vi "optagefrekvenssignal0.8.vi"() -> ()   [LabVIEW 2014]
uses:
  <vilib>/measure/maspectr.llb/FFT Power Spectrum and PSD for 1 Chan.vi
  <vilib>/Utility/file.llb/Write To Spreadsheet File (DBL).vi
  <vilib>/measure/NI_MAPro.lvlib
panel:
  out "Resonansfrekvens, første 10 målinger":dbl[](array[numeric])
  in  "Tid(sek)":dbl
  out "Resonansfrekvens af kammer med objekt":dbl
  out "FFT af lydsignal":dbl[](graph)
  out "Lydsignal":waveform(dbl)(graph)
  # "Gennemsnit"
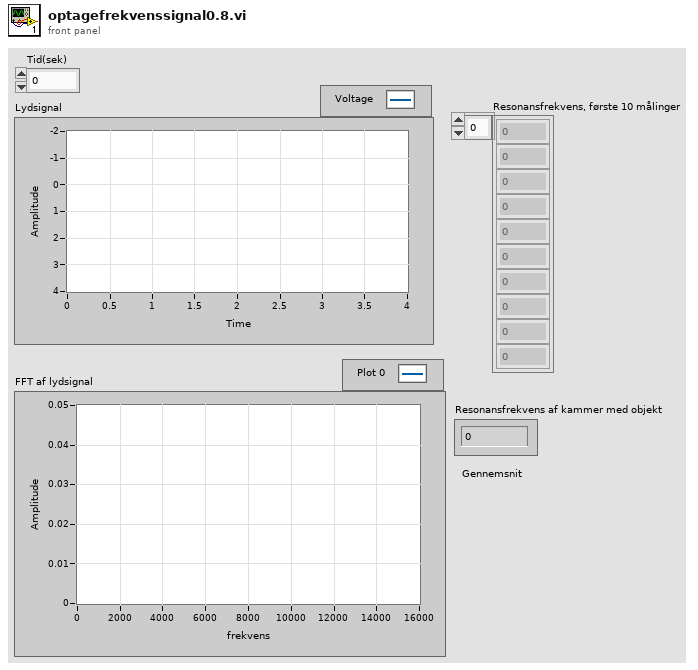
[diagram p1: front panel]
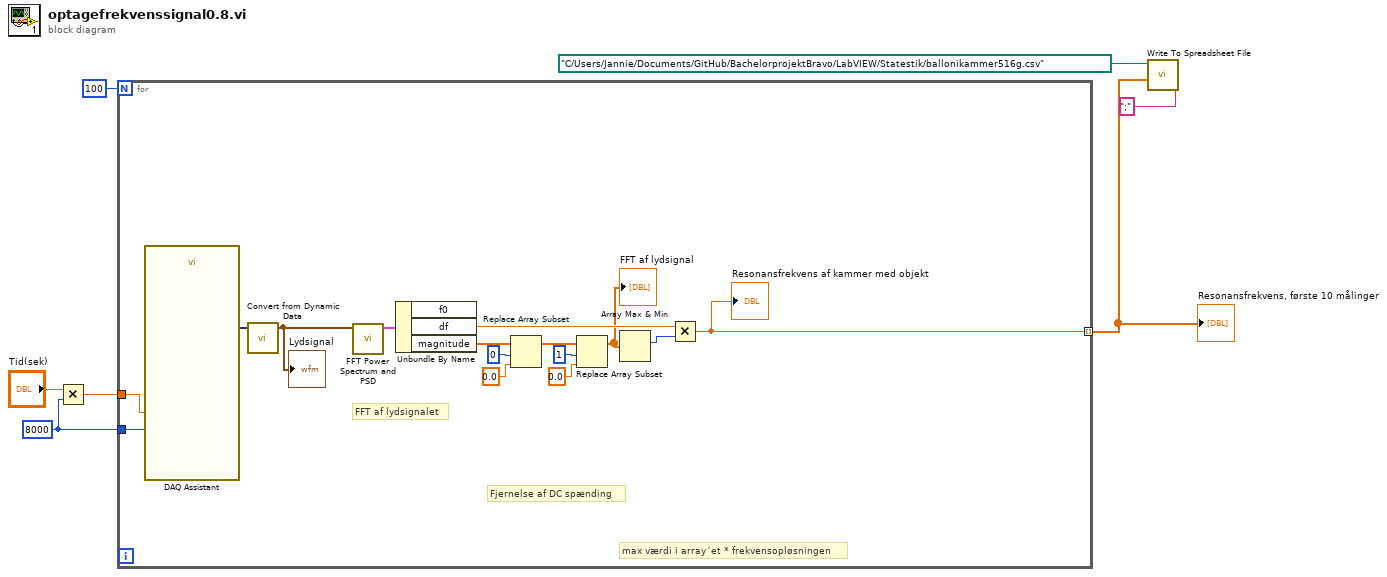
[diagram p0: block diagram]
diagram:
  w3 = 8000
  n1 = Multiply(x="Tid(sek)", y=w3) -> (x*y=w2:dbl)
  n2 = for {
    N: 100 -> [_]
    tunnel: [w12] -> w1 mode=indexing
    tunnel: w3 -> [w10]
    tunnel: w2 -> [w9]
    # "max værdi i array´et * frekvensopløsningen"
    # "Fjernelse af DC spænding"
    # "FFT af lydsignalet"
    n3 = call "DAQ Assistant"("rate"=w10, "number of samples"=w9) -> ("data"=w8:dynamicdata)  [unwired: 15 in, 2 out]
    n4 = call "Convert from Dynamic Data"("Dynamic Data Type"=w8) -> ("Waveform"=w11:waveform(dbl))  [unwired: 3 in]
    "Lydsignal" <- w11
    n5 = call-poly <vilib>:"FFT Power Spectrum and PSD.vi"("time signal"=w11) -> ("Power Spectrum / PSD"=w15:cluster{"f0":dbl, "df":dbl, "magnitude":dbl[]})  [unwired: 7 in, 3 out]
    n6 = Unbundle By Name(w15) -> ("df"=w16:dbl, "magnitude"=w14:dbl[])  [unwired: 1 out]
    n7 = Replace Array Subset(array=w14, new element=0.0 ("new element/subarray"), index=0) -> (w20:dbl[])
    n8 = Replace Array Subset(array=w20, new element=0.0 ("new element/subarray"), index=1) -> (w13:dbl[])
    "FFT af lydsignal" <- w13
    n9 = Array Max & Min(array=w13) -> (max index (indices)=w17:i32)  [unwired: 3 out]
    n10 = Multiply(x=w16, y=w17) -> (x*y=w12:dbl)
    "Resonansfrekvens af kammer med objekt" <- w12
  }
  "Resonansfrekvens, første 10 målinger" <- w1
  n11 = call-poly <vilib>:"Write To Spreadsheet File.vi"("delimiter (\\t)"=";" ("delimiter (\\t)"), "1D data"=w1, "file path (dialog if empty)"=path "C:/Users/Jannie/Documents/GitHub/BachelorprojektBravo/LabVIEW/Statestik/ballonikammer516g.csv") -> ()  [unwired: 5 in, 1 out]
